vi "Get Selected VIs.vi"(7 "error in":errorcluster, 8 "Selected Indexes":i32[](array[numeric]), 10 "Listbox Contents":T1) -> (0 "error out":errorcluster, 3 "Selected Listbox Contents":T1)   [LabVIEW 2020]
uses:
  <vilib>/SourceOnly/NI_SourceOnly_CollectionOfVIsAndLibraries.ctl
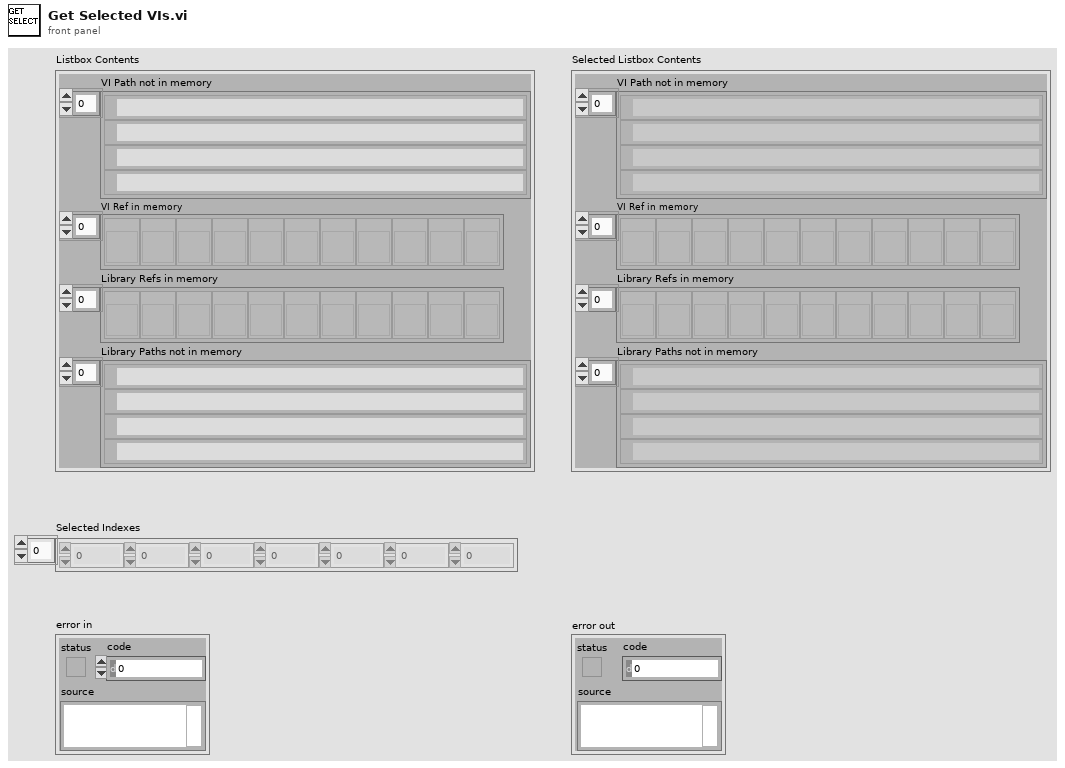
[diagram p1: front panel]
types:
  T1 = typedef "NI_SourceOnly_CollectionOfVIsAndLibraries.ctl" = cluster{"VI Path not in memory":path[], "VI Ref in memory":refnum<vi>[], "Library Refs in memory":refnum<vi>[], "Library Paths not in memory":path[]}
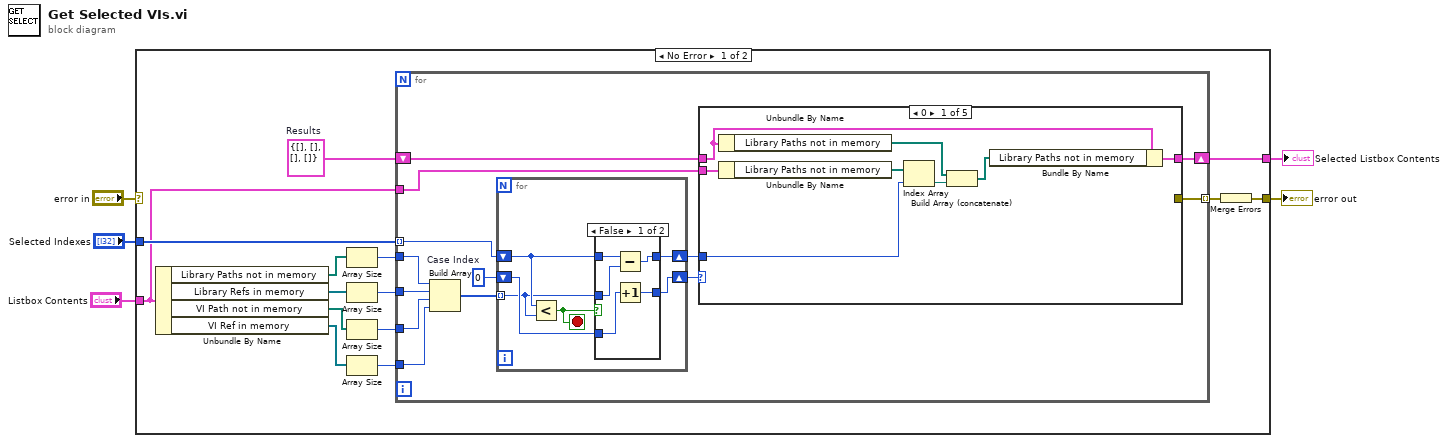
[diagram p0: block diagram]
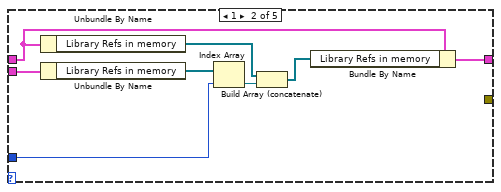
[diagram p2: hidden frame]
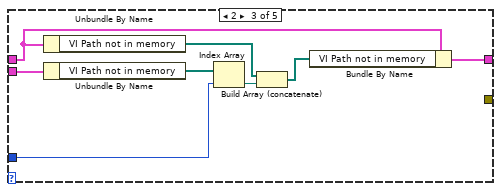
[diagram p3: hidden frame]
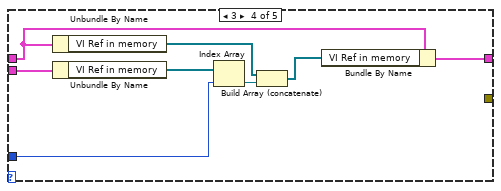
[diagram p4: hidden frame]
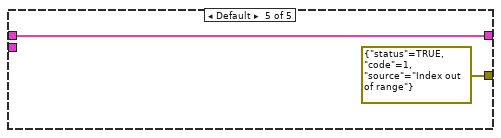
[diagram p5: hidden frame]
diagram:
  n1 = case shown="No Error" "error in" {
    selector: "error in" -> [_ w80]
    tunnel: [w19 w80] -> w4
    tunnel: "Selected Indexes" -> [w18 _]
    tunnel: "Listbox Contents" -> [w8 _]
    tunnel: [w7 _] -> w1
    frame No Error {
      w17 = T1 {"VI Path not in memory"=[], "VI Ref in memory"=[], "Library Refs in memory"=[], "Library Paths not in memory"=[]}  # Results
      n2 = Unbundle By Name(w8) -> ("Library Paths not in memory"=w16:path[], "Library Refs in memory"=w15:refnum<vi>[], "VI Path not in memory"=w14:path[], "VI Ref in memory"=w13:refnum<vi>[])
      n3 = Array Size(array=w16) -> (size(s)=w12:i32)
      n4 = Array Size(array=w15) -> (size(s)=w11:i32)
      n5 = Array Size(array=w14) -> (size(s)=w10:i32)
      n6 = Array Size(array=w13) -> (size(s)=w9:i32)
      n7 = for {
        tunnel: w18 -> [w25] mode=indexing
        shift-right: [w21] -> w7
        shift-left: w17 -> [w20]
        tunnel: w12 -> [w31]
        tunnel: w11 -> [w30]
        tunnel: w10 -> [w29]
        tunnel: w9 -> [w28]
        tunnel: w8 -> [w22]
        tunnel: [w32] -> w6 mode=indexing
        w26 = 0  # Case Index
        n8 = Build Array(w31, w30, w29, w28) -> (w27:i32[])
        n9 = for {
          tunnel: w27 -> [w67] mode=indexing
          shift-right: [w68] -> w24
          shift-left: w26 -> [w71]
          shift-right: [w70] -> w23
          shift-left: w25 -> [w69]
          stop <- w72 stop-if-true
          n10 = Less?(x=w69, y=w67) -> (x < y?=w72:bool)
          n11 = case shown="False" w72 {
            tunnel: w71 -> [w75 w78]
            tunnel: [w77 w79] -> w70
            tunnel: w69 -> [w76 w79]
            tunnel: [w73 w78] -> w68
            tunnel: w67 -> [w74 _]
            frame False {
              n12 = Subtract(x=w76, y=w74) -> (x-y=w77:i32)
              n13 = Increment(x=w75) -> (x+1=w73:i32)
            }
            frame True {
            }
          }
        }
        n14 = case shown="0" w24 {
          tunnel: w22 -> [w40 w48 w56 w64 _]
          tunnel: w23 -> [w38 w46 w54 w62 _]
          tunnel: [w33 w41 w49 w57 w65] -> w21
          tunnel: w20 -> [w34 w45 w53 w61 w65]
          tunnel: [_ _ _ _ errorcluster {"status"=TRUE, "code"=1, "source"="Index out of range"} ("error IO")] -> w32
          frame 0 {
            n15 = Unbundle By Name(w34) -> ("Library Paths not in memory"=w37:path[])
            n16 = Unbundle By Name(w40) -> ("Library Paths not in memory"=w39:path[])
            n17 = Index Array(array=w39, index=w38) -> (element=w35:path)
            n18 = Build Array (concatenate)(w37, w35) -> (w36:path[])
            n19 = Bundle By Name(cluster=w34, "Library Paths not in memory"=w36) -> (w33:T1)
          }
          frame 1 {
            n20 = Unbundle By Name(w45) -> ("Library Refs in memory"=w44:refnum<vi>[])
            n21 = Unbundle By Name(w48) -> ("Library Refs in memory"=w47:refnum<vi>[])
            n22 = Index Array(array=w47, index=w46) -> (element=w42:refnum<vi>)
            n23 = Build Array (concatenate)(w44, w42) -> (w43:refnum<vi>[])
            n24 = Bundle By Name(cluster=w45, "Library Refs in memory"=w43) -> (w41:T1)
          }
          frame 2 {
            n25 = Unbundle By Name(w53) -> ("VI Path not in memory"=w52:path[])
            n26 = Unbundle By Name(w56) -> ("VI Path not in memory"=w55:path[])
            n27 = Index Array(array=w55, index=w54) -> (element=w50:path)
            n28 = Build Array (concatenate)(w52, w50) -> (w51:path[])
            n29 = Bundle By Name(cluster=w53, "VI Path not in memory"=w51) -> (w49:T1)
          }
          frame 3 {
            n30 = Unbundle By Name(w61) -> ("VI Ref in memory"=w60:refnum<vi>[])
            n31 = Unbundle By Name(w64) -> ("VI Ref in memory"=w63:refnum<vi>[])
            n32 = Index Array(array=w63, index=w62) -> (element=w58:refnum<vi>)
            n33 = Build Array (concatenate)(w60, w58) -> (w59:refnum<vi>[])
            n34 = Bundle By Name(cluster=w61, "VI Ref in memory"=w59) -> (w57:T1)
          }
          frame Default {
          }
        }
      }
      n35 = Merge Errors(w6) -> (w19:errorcluster)
    }
    frame Error {
    }
  }
  "error out" <- w4
  "Selected Listbox Contents" <- w1
